vi "Clone.vi"(8 "error in (no error)":errorcluster, 11 "BaseDriver in":refnum<class "BaseDriver.lvclass">) -> (0 "error out":errorcluster, 3 "BaseDriver out":refnum<class "BaseDriver.lvclass">)   [LabVIEW 2013, in "BaseDriver.lvclass"]
doc: "Initializes a new instance of the driver. Use to create a clone of the driver to start in parallel as the original"
uses:
  BaseDriver.lvclass
  BaseDriver.lvclass/BaseDriver.ctl
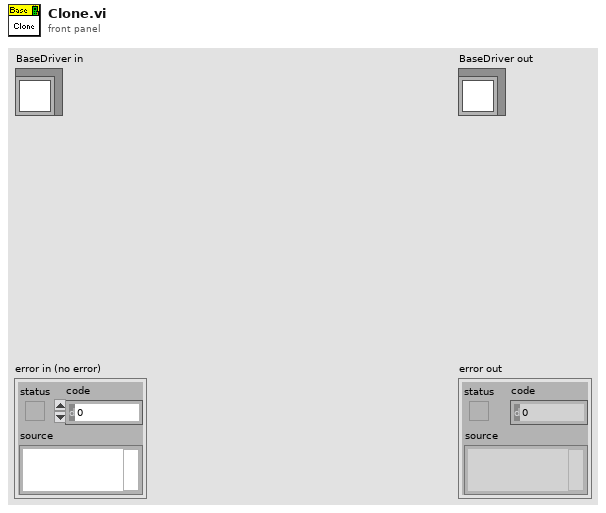
[diagram p1: front panel]
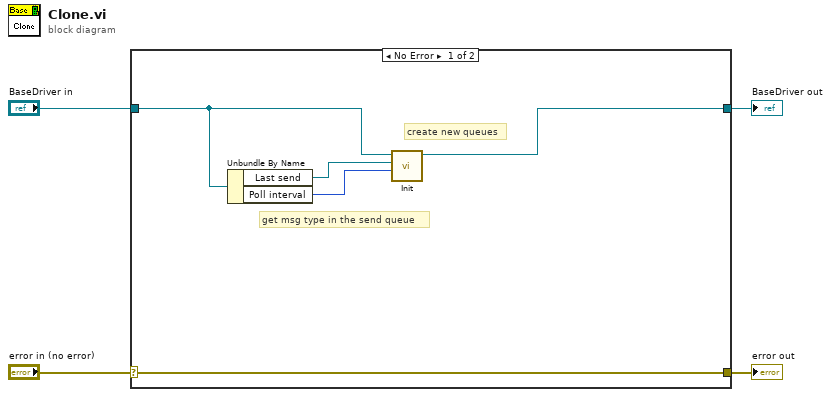
[diagram p0: block diagram]
diagram:
  n1 = case shown="No Error" "error in (no error)" {
    selector: "error in (no error)" -> [w9 w11]
    tunnel: [w9 w11] -> w3
    tunnel: [w8 w10] -> w1
    tunnel: "BaseDriver in" -> [w7 w10]
    frame No Error {
      # "create new queues"
      # "get msg type in the send queue"
      n2 = Unbundle By Name(w7) -> ("Last send"=w6:refnum<class "BaseMessage.lvclass">, "Poll interval"=w5:i32)
      n3 = call "Init.vi"("Poll interval"=w5, "Message type"=w6, "BaseDriver in"=w7) -> ("BaseDriver out"=w8:refnum<class "BaseDriver.lvclass">)  [unwired: 6 in, 2 out]
    }
    frame Error {
    }
  }
  "error out" <- w3
  "BaseDriver out" <- w1
